vi "copy data to identical cluster.vi"(9 "Guest Clust Refnum":refnum<vi>, 11 "Host Clust Refnum":refnum<vi>) -> ()   [LabVIEW 2015]
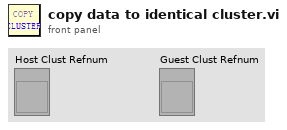
[diagram p1: front panel]
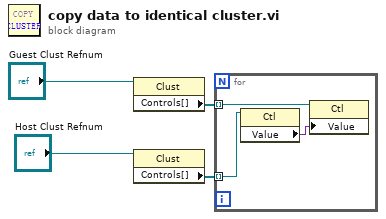
[diagram p0: block diagram]
diagram:
  n1 = property class="Clust"(reference="Guest Clust Refnum") -> ("Controls[]"=w1:refnum<vi>[])  [unwired: 1 in, 2 out]
  n2 = property class="Clust"(reference="Host Clust Refnum") -> ("Controls[]"=w2:refnum<vi>[])  [unwired: 1 in, 2 out]
  n3 = for {
    tunnel: w2 -> [w7] mode=indexing
    tunnel: w1 -> [w6] mode=indexing
    n4 = property class="Ctl"(reference=w7) -> ("Value"=w5:variant)  [unwired: 1 in, 2 out]
    n5 = property class="Ctl"(reference=w6, "Value"=w5) -> ()  [unwired: 1 in, 2 out]
  }
